vi "oct_ui.vi"() -> ()   [LabVIEW 2012]
uses:
  <vilib>/Platform/TimedLoop/XDataNode/timing_clust.ctl
  <vilib>/Platform/TimedLoop/XDataNode/nitl_modes.ctl
  <vilib>/Platform/TimedLoop/XDataNode/wakeup.ctl
  stimulus.ctl
  injection_point.ctl
  <vilib>/Analysis/3filter.llb/Filter Passband Type.ctl
  initialization/micron_globals.vi
  <vilib>/Analysis/3filter.llb/Zero Phase Filter (Cascade, DBL).vi
  <vilib>/Analysis/Matrix/Numeric/Conversions/Array To Matrix.vi
  <vilib>/Analysis/Matrix/Numeric/Conversions/Array To Matrix - RA.vi
  <vilib>/Analysis/7linalg.llb/Create Special Real Matrix.vi
  <vilib>/Platform/TimedLoop/XDataNode/XDataNode.xnode
  <vilib>/Platform/TimedLoop/XDataNode/XDNodeRunTimeDep.lvlib
  <vilib>/measure/NI_MABase.lvlib
  <vilib>/Analysis/NI_AALBase.lvlib
  <vilib>/Analysis/NI_AALPro.lvlib
panel:
  in  "stop":bool
  in  "Amplitude":dbl=500.0 min=0.0 max=2000.0 step=100.0 format="%#_6p"
  in  "Bandwidth":dbl=10.0 format="%0.3f"
  in  "Frequency":dbl=2.5
  in  "RCM offset":sgl(slide)=16.020409 scale=30.0..5.0 scale format="%#.0f"
  in  "Scan rotation":dbl(slide)=-5.10702591327572e-15 min=-90.0 max=90.0 scale=-90.0..90.0
  # "OCT user interface"
  # "Scan parameters"
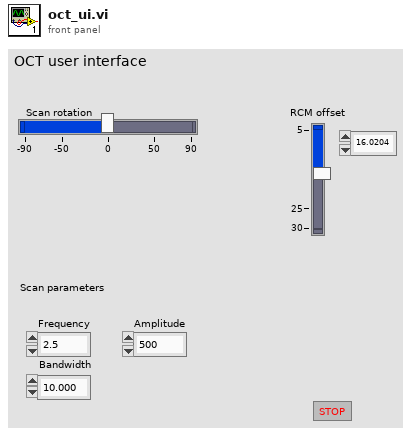
[diagram p1: front panel]
types:
  T1 = typedef "ui_override_opts.ctl" = cluster{"Triggering":bool, "Parameters":bool, "Stimulus":bool, "Calibration":bool, "Modes":bool}
  T2 = typedef "XDNodeRunTimeDep.lvlib/timing_clust.ctl" = cluster{"Expected End [f-1]":u64, "Actual End [f-1]":u64, "Finished Late? [f-1]":bool, "Expected End [i-1]":u64, "Actual End [i-1]":u64, "Finished Late? [i-1]":bool, "Expected Start [i]":u64, "Actual Start [i]":u64, "Expected Start [f]":u64, "Actual Start [f]":u64, "Source Name":string, "Structure Name":string, "Period":i64, "Deadline":i64, "Offset":i64, "Start":i64, "Priority":i32, "Timeout":i32, "Mode":T3, "Wakeup Reason":T4, "Error":errorcluster, "Source Type":string, "Secondary Source Type":string, "Global End Time":u64, "Global Start Time":u64, "Frame Duration":u64, "Iteration Duration":u64, "Assigned CPU":i32, "I/O Scan Engine Mode":u32}
  T3 = typedef "XDNodeRunTimeDep.lvlib/nitl_modes.ctl" = enum32{"No Change", "Process missed periods, maintain original phase", "Discard missed periods, maintain original phase", "Process missed periods, ignore original phase", "Discard missed periods, ignore original phase"}
  T4 = typedef "XDNodeRunTimeDep.lvlib/wakeup.ctl" = enum32{"Normal", "Aborted", "Asynchronous wakeup", "Timing source error", "Timed loop error", "Timeout"}
  T5 = typedef "NI_AALBase.lvlib/Filter Passband Type.ctl" = enum32{"Lowpass", "Highpass", "Bandpass", "Bandstop"}
  T6 = typedef "stimulus.ctl" = cluster{"Type":enum16{"Off", "Step", "Sine", "Triangle", "Arbitrary"}, "Phase":dbl, "Amplitude":sgl[], "Injection point":T7, "Closed loop":bool, "Offset":sgl[], "Tip -> world":bool, "Frequency":dbl, "Length":dbl}
  T7 = typedef "injection_point.ctl" = enum16{"Total pose", "V limiter", "Goal ", "Link position", "KF link position", "Inverse kin", "Link goal", "Link error", "Controller", "Output", "Drive", "Light"}
  T8 = typedef "Micron params.ctl" = cluster{"Stimulus":T6, "Goal Filter A":T9, "Mode controls":T10, "Manipulator type":enum16{"Current piezo", "Voltage piezo"}, "Manipulator calibration":T11, "Network":T13, "Goal Filter B":T9, "Cancellation":T14, "Transition time":sgl, "Estimation":T16}
  T9 = typedef "goal_loop_parms.ctl" = cluster{"Speedup max":sgl, "Speedup thresh":sgl, "Speedup nonlin":sgl, "Filters":cluster{"Lower Fc":sgl, "Lower Q":sgl, "Scale factor":sgl, "Upper Fc":sgl, "Upper Q":sgl, "V limit":sgl, "V limit range":sgl}[]}
  T10 = typedef "mode_conrols.ctl" = cluster{"Hold":bool, "Cancellation":bool, "Goal filter":bool, "Trigger":bool}
  T11 = typedef "manipulator_cal.ctl" = cluster{"Tool offsets":sgl[][], "Tip light calibration":T12, "Handle light calibration":T12, "Base pivots":sgl[][], "Output pivots":sgl[][], "Length center":sgl, "Workspace height":sgl[], "Workspace diameter":sgl[], "Linearization":sgl[][], "Stack travel":sgl, "Saturation pos":sgl, "Inverse filters":cluster{"filter structure":enum32{"IIR 2nd Order", "IIR 4th Order"}, "Reverse Coefficients":dbl[], "Forward Coefficients":dbl[]}[]}
  T12 = typedef "probe_calibration.ctl" = sgl[][]
  T13 = typedef "network_params.ctl" = cluster{"Remote Host":string, "Send Status":bool, "Send Port":u16, "Recv Commands":bool, "Recv Port":u16}
  T14 = typedef "sq_control_params.ctl" = cluster{"KP":T15, "KI":sgl, "KD":T15, "Max vel":sgl, "Max acc":sgl, "Int error limit":sgl, "RCM gain":sgl, "Bypass":bool, "Degraded gain":sgl}
  T15 = typedef "decoupled_gain.ctl" = cluster{"XY":sgl, "Rxy":sgl, "Z":sgl, "Rz":sgl}
  T16 = typedef "estimation_controls.ctl" = cluster{"Link":cluster{"Measure noise":dbl[], "Process noise":dbl[], "Alt process noise":dbl[], "Alt turnoff cycles":i32, "Innovation limit":dbl[], "Residue threshold":dbl, "Enable":bool}, "Handle":cluster{"Measure noise":dbl[], "Process noise":dbl[], "State limits":dbl[], "Innovation limit":dbl[], "Prediction Lookahead":sgl, "Enable":bool}}
  T17 = typedef "NI_Matrix.lvlib/RealMatrix.ctl" = dbl[][]
  T18 = cluster{"filter structure":enum32{"IIR 2nd Order", "IIR 4th Order"}, "Reverse Coefficients":dbl[], "Forward Coefficients":dbl[]}
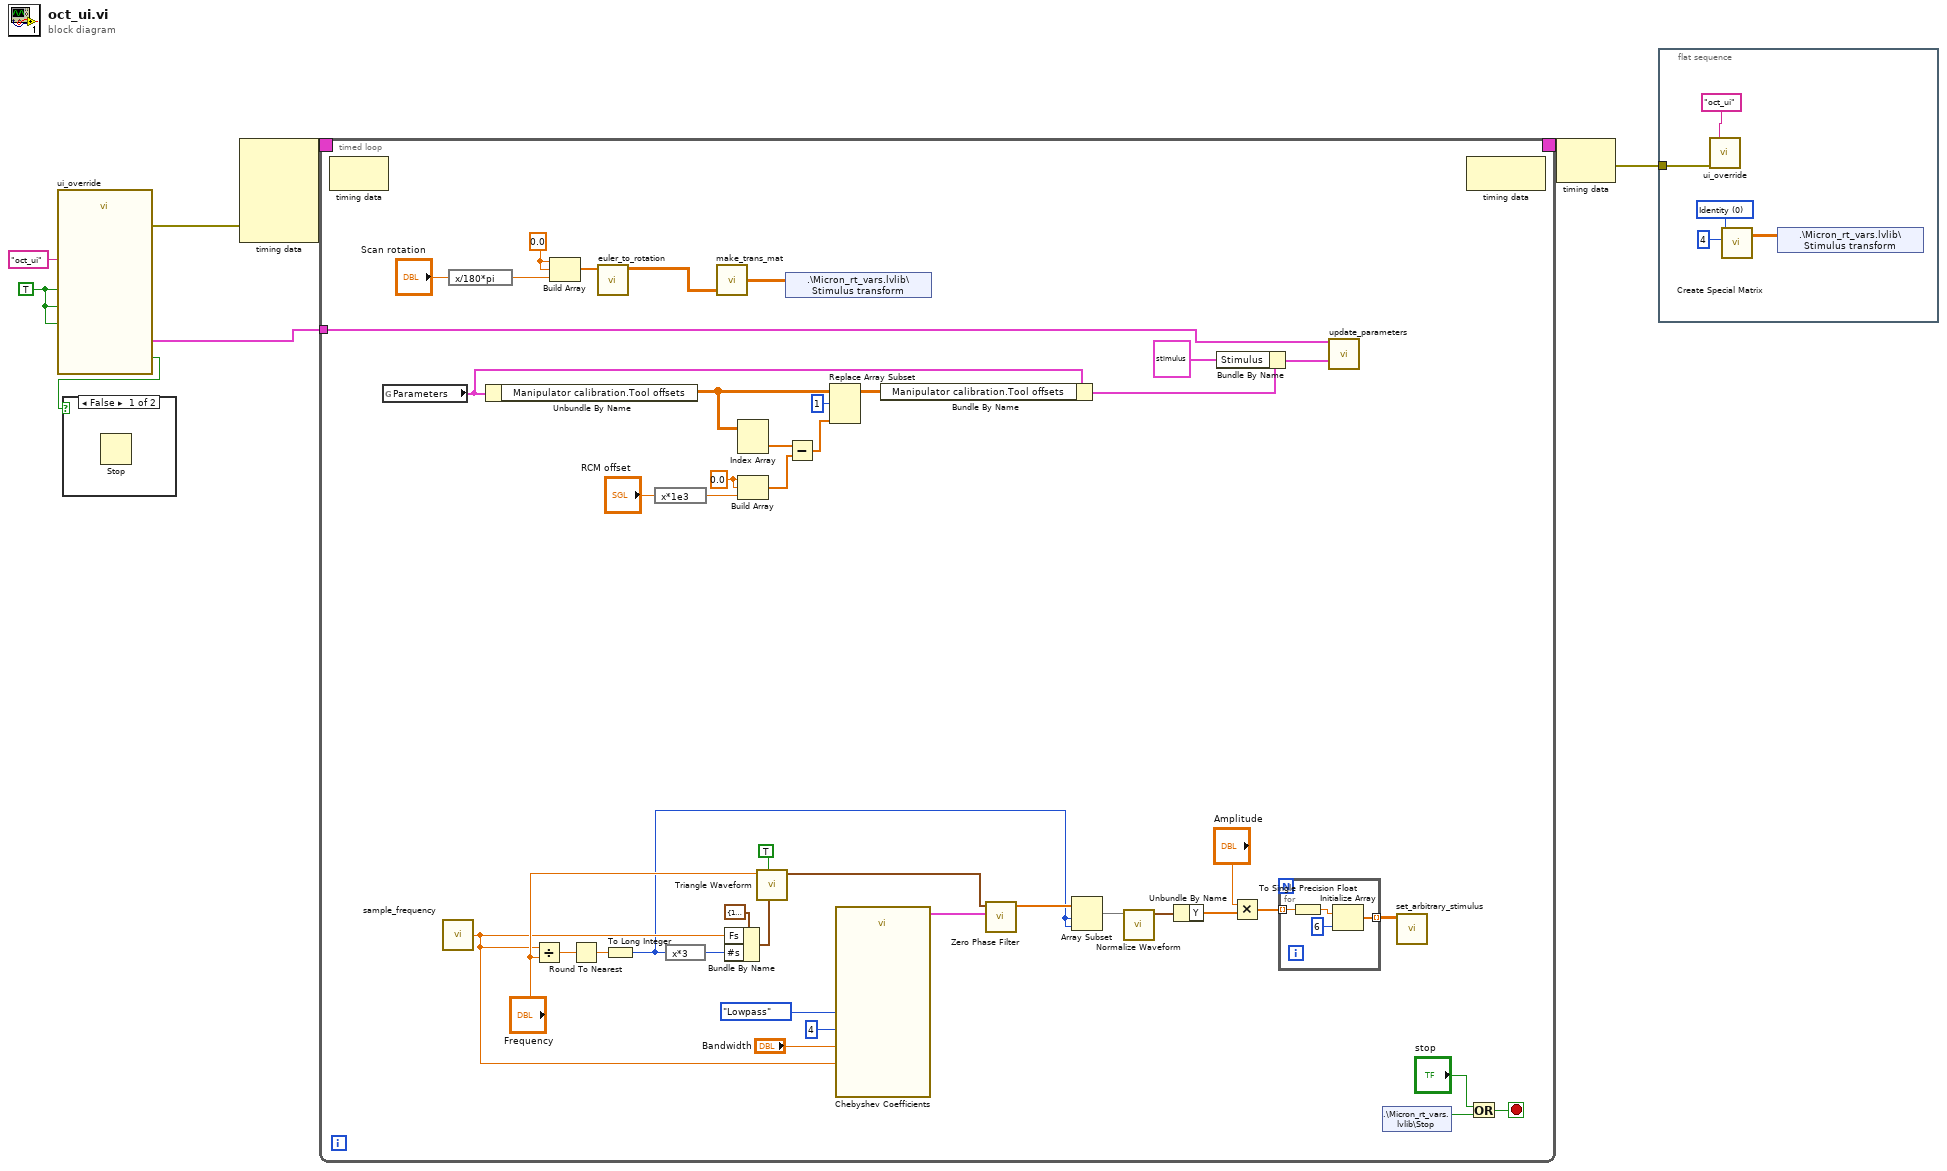
[diagram p0: block diagram]
diagram:
  w4 = TRUE ("All or nothing")
  n1 = call "ui_override.vi"("VI name"="oct_ui", "Stimulus"=w4, "Calibration"=w4, "All or nothing"=w4) -> ("Override"=w2:T1, "Got all"=w3:bool, "error out"=w6:errorcluster)  [unwired: 9 in]
  n2 = case shown="False" w3 {
    frame False {
      n3 = Stop() -> ()  [unwired: 1 in]
    }
    frame True {
    }
  }
  n4 = node-c288(w6) -> (w8:T2)  [unwired: 4 in]
  n5 = timed-loop {
    timing: w8 -> [_]
    timing-out: [_] -> w7
    tunnel: w2 -> [w12]
    stop <- w9 stop-if-true
    w43 = sgl 0.0 ("element")
    w52 = 0.0 ("element")
    n6 = node-c288() -> ()  [unwired: 1 in, 1 out]
    n7 = global read "micron_globals.vi" "Parameters"() -> (w40:T8)
    n8 = call "sample_frequency.vi"() -> ("Sample frequency"=w29:dbl)
    n9 = expression code="x/180*pi"("Scan rotation") -> (w47:dbl)
    n10 = Unbundle By Name(w40) -> ("Manipulator calibration.Tool offsets"=w45:sgl[][])
    n11 = Divide(x=w29, y="Frequency") -> (x/y=w34:dbl)
    n12 = Build Array(w52, w52, w47) -> (w51:dbl[])
    n13 = Round To Nearest(number=w34) -> (nearest integer value=w20:dbl)
    n14 = call "euler_to_rotation.vi"("Theta XYZ"=w51) -> ("Rotation"=w50:T17)  [unwired: 10 in]
    n15 = To Long Integer(number=w20) -> (32bit integer=w19:i32)
    n16 = expression code="x*1e3"("RCM offset") -> (w37:sgl)
    n17 = expression code="x*3"(w19) -> (w22:i32)
    n18 = call "make_trans_mat.vi"("Rotation"=w50) -> ("Transform"=w49:T17)  [unwired: 4 in]
    n19 = Bundle By Name(cluster=cluster{"Fs":dbl, "#s":dbl} {"Fs"=1000.0, "#s"=1000.0} ("sampling info"), "Fs"=w29, "#s"=w22) -> (w32:cluster{"Fs":dbl, "#s":dbl})
    n20 = Index Array(array=w45) -> (element=w44:sgl[])  [unwired: 2 in]
    n21 = Build Array(w43, w43, w37) -> (w42:sgl[])
    n22 = call <vilib>:"Triangle Waveform.vi"("sampling info"=w32, "reset signal"=TRUE, "frequency"="Frequency") -> ("signal out"=w24:waveform(dbl))  [unwired: 7 in, 1 out]
    n23 = shared-variable ".\\Micron_rt_vars.lvlib\\Stimulus transform"(w49) -> ()  [unwired: 2 out]
    n24 = Subtract(x=w44, y=w42) -> (x-y=w41:sgl[])
    n25 = Replace Array Subset(array=w45, new element=w41, index (row)=1) -> (w39:sgl[][])  [unwired: 1 in]
    n26 = call <vilib>:"Chebyshev Coefficients.vi"("order"=4, "filter type"=Filter_Passband_Type."Lowpass", "low cutoff freq: fl"="Bandwidth", "sampling freq: fs"=w29) -> ("IIR Filter Cluster"=w25:T18)  [unwired: 6 in, 1 out]
    n27 = Bundle By Name(cluster=w40, "Manipulator calibration.Tool offsets"=w39) -> (w13:T8)
    n28 = call-poly <vilib>:"Zero Phase Filter.vi"("IIR Filter Cluster"=w25, "X"=w24) -> ("Filtered X"=w21:dbl[])  [unwired: 8 in, 1 out]
    n29 = Array Subset(array=w21, index=w19, length=w19) -> (w18:dbl[])
    n30 = call <vilib>:"Normalize Waveform.vi"("waveform in"=w18) -> ("normalized waveform"=w15:waveform(dbl))  [unwired: 7 in, 3 out]
    n31 = Unbundle By Name(w15) -> ("Y"=w14:dbl[])
    n32 = Bundle By Name(cluster=w13, "Stimulus"=T6 {"Type"=enum."Arbitrary", "Phase"=0.0, "Amplitude"=[1.0, 0.0, 0.0, 0.0, 0.0, 0.0], "Injection point"=enum."Goal ", "Closed loop"=TRUE, "Offset"=[0.0, 0.0, 0.0, 0.0, 0.0, 0.0], "Tip -> world"=TRUE, "Frequency"=2.5, "Length"=0.0}) -> (w36:T8)
    n33 = Multiply(x="Amplitude", y=w14) -> (x*y=w16:dbl[])
    n34 = for {
      tunnel: w16 -> [w54] mode=indexing
      tunnel: [w55] -> w23 mode=indexing
      n35 = To Single Precision Float(number=w54) -> (single precision float=w53:sgl)
      n36 = Initialize Array(w53, 6 ("dimension size")) -> (w55:sgl[])
    }
    n37 = call "update_parameters.vi"("Modify"=w12, "Parameters"=w36) -> ()  [unwired: 12 in, 2 out]
    n38 = shared-variable ".\\Micron_rt_vars.lvlib\\Stop"() -> (w10:bool)  [unwired: 2 out]
    n39 = call "set_arbitrary_stimulus.vi"("New stimulus"=w23) -> ()  [unwired: 11 in]
    n40 = node-c288() -> ()  [unwired: 1 in, 1 out]
    n41 = Or(x="stop", y=w10) -> (x .or. y?=w9:bool)
  }
  n42 = node-c288(w7) -> (w1:errorcluster)
  n43 = flat-sequence {
    tunnel: w1 -> [w62]
    frame #0 {
      w61 = 0 items=["Identity", "Diagonal", "Toeplitz", "Vandermonde", "Companion", "Hankel", "Hadamard", "Wilkinson", "Hilbert", "Inverse Hilbert", "Rosser", "Pascal"] ("matrix type")
      n44 = call "ui_override.vi"("VI name"="oct_ui", "error in"=w62) -> ()  [unwired: 11 in, 3 out]
      n45 = call-poly <vilib>:"Create Special Matrix.vi"("matrix type"=w61, "matrix size"=4) -> ("Special Matrix"=w60:T17)  [unwired: 3 in, 1 out]
      n46 = shared-variable ".\\Micron_rt_vars.lvlib\\Stimulus transform"(w60) -> ()  [unwired: 2 out]
    }
  }
